vi "setAttribute_ArgumentList.vi"(7 "object":string, 8 "error in (no error)":errorcluster, 9 "argument list in":T1[](array[typedef]), 10 "attribute":string, 11 "LabVIEW-Python-Interface in":refnum<class "PyLVi.lvclass">) -> (0 "error out":errorcluster, 1 "return list":T1[](array[typedef]), 3 "LabVIEW-Python-Interface out":refnum<class "PyLVi.lvclass">)   [LabVIEW 2016, in "PyLVi.lvlib" / "PyLVi.lvclass"]
uses:
  PyLVi.lvclass
  Controls/ArgumentStructure.ctl
  Controls/DescriptorStructure.ctl
  Controls/AttributeStructure.ctl
panel:
  out "return message":string
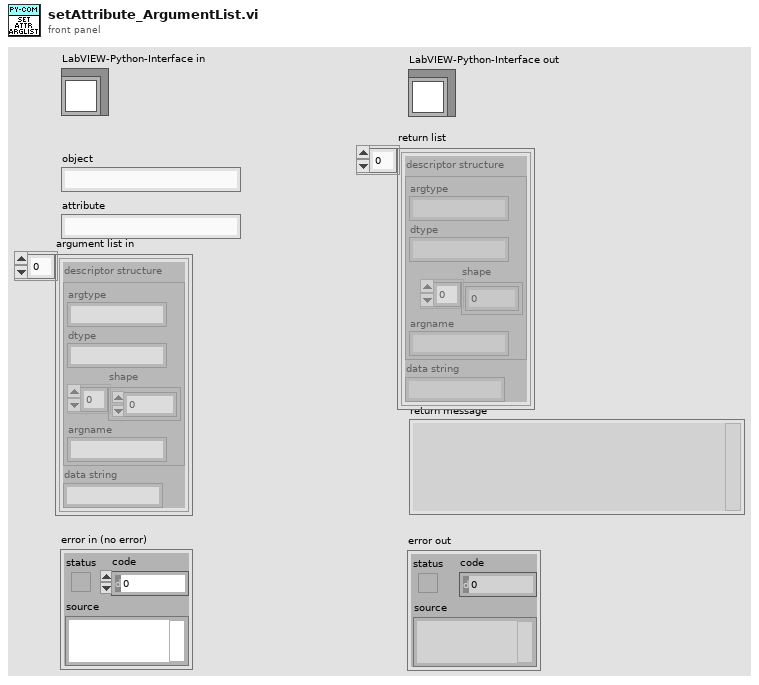
[diagram p1: front panel]
types:
  T1 = typedef "PyLVi.lvlib/PyLVi.lvclass/ArgumentStructure.ctl" = cluster{"descriptor structure":T2, "data string":string}
  T2 = typedef "PyLVi.lvlib/PyLVi.lvclass/DescriptorStructure.ctl" = cluster{"argtype":string, "dtype":string, "shape":u32[], "argname":string}
  T3 = typedef "PyLVi.lvlib/PyLVi.lvclass/AttributeStructure.ctl" = cluster{"obj":string, "attr":string, "access":string}
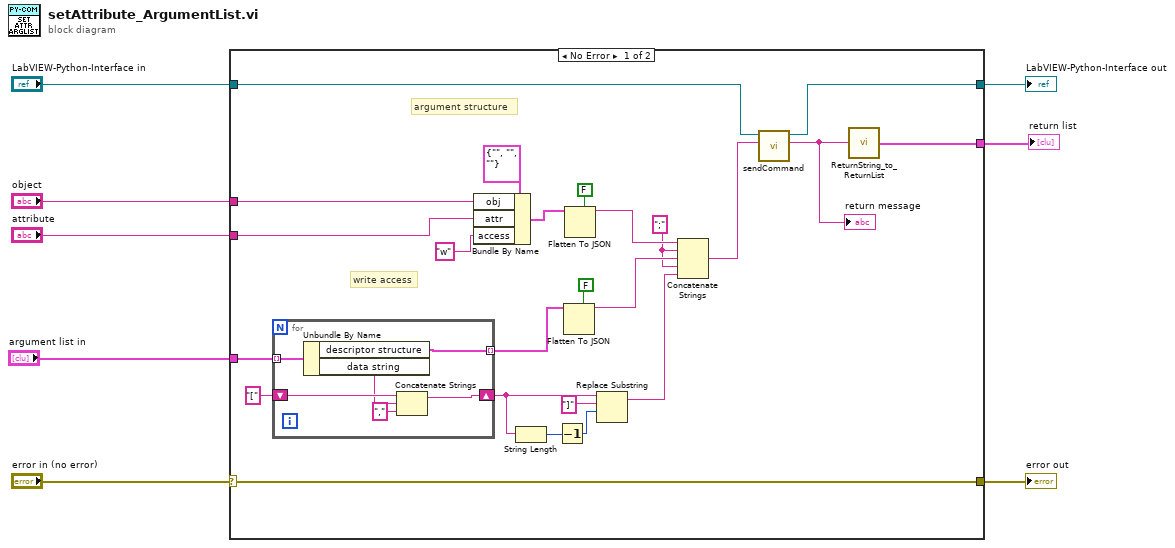
[diagram p0: block diagram]
diagram:
  n1 = case shown="No Error" "error in (no error)" {
    selector: "error in (no error)" -> [w32 w39]
    tunnel: [w32 w39] -> w7
    tunnel: [w30 w40] -> w5
    tunnel: "LabVIEW-Python-Interface in" -> [w31 w40]
    tunnel: "object" -> [w29 _]
    tunnel: "attribute" -> [w28 _]
    tunnel: "argument list in" -> [w20 _]
    tunnel: [w17 _] -> w1
    frame No Error {
      w22 = ";" ("string")
      # "write access"
      # "argument structure"
      n2 = for {
        tunnel: w20 -> [w38] mode=indexing
        tunnel: [w37] -> w19 mode=indexing
        shift-right: [w36] -> w14
        shift-left: "[" ("string") -> [w35]
        n3 = Unbundle By Name(w38) -> ("descriptor structure"=w37:T2, "data string"=w34:string)
        n4 = Concatenate Strings(w35, w34, "," ("string")) -> (w36:string)
      }
      n5 = Bundle By Name(cluster=T3 {"obj"="", "attr"="", "access"=""} ("attribute command structure"), "obj"=w29, "attr"=w28, "access"="w") -> (w27:T3)
      n6 = String Length(string=w14) -> (length=w13:i32)
      n7 = Decrement(x=w13) -> (x-1=w12:i32)
      n8 = Flatten To JSON(enable LabVIEW extensions? (T)=FALSE, anything=w19) -> (JSON string=w23:string)  [unwired: 1 in, 1 out]
      n9 = Flatten To JSON(enable LabVIEW extensions? (T)=FALSE, anything=w27) -> (JSON string=w25:string)  [unwired: 1 in, 1 out]
      n10 = Replace Substring(3:w12, 4:"]" ("string"), 5:w14) -> (1:w11:string)  [unwired: 1 in, 1 out]
      n11 = Concatenate Strings(w25, w22, w23, w22, w11) -> (w21:string)
      n12 = call "sendCommand.vi"("command"=w21, "LabVIEW-Python-Interface in"=w31) -> ("data"=w18:string, "LabVIEW-Python-Interface out"=w30:refnum<class "PyLVi.lvclass">)  [unwired: 6 in, 2 out]
      "return message" <- w18
      n13 = call "ReturnString_to_ReturnList.vi"("return string"=w18) -> ("return list"=w17:T1[])  [unwired: 3 in, 1 out]
    }
    frame Error {
    }
  }
  "error out" <- w7
  "LabVIEW-Python-Interface out" <- w5
  "return list" <- w1
